vi "push.vi"() -> ()   [LabVIEW 2010]
panel:
  in  "stop":bool
  in  "OME string":string
  in  "notebook string":string
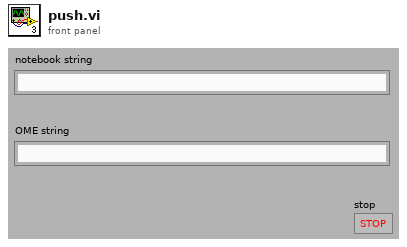
[diagram p1: front panel]
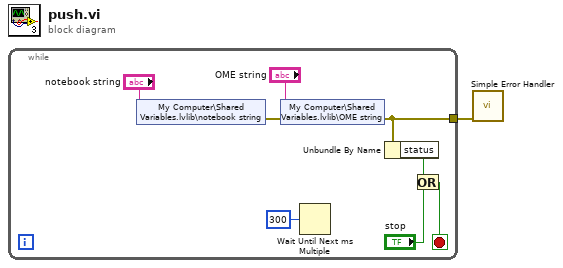
[diagram p0: block diagram]
diagram:
  n1 = while {
    tunnel: [w2] -> w1
    stop <- w3 stop-if-true
    n2 = shared-variable "My Computer\\Shared Variables.lvlib\\notebook string"("notebook string") -> (error out=w6:errorcluster)  [unwired: 1 in]
    n3 = shared-variable "My Computer\\Shared Variables.lvlib\\OME string"("OME string", error in=w6) -> (error out=w2:errorcluster)
    n4 = Wait Until Next ms Multiple(millisecond multiple=u32 300) -> ()  [unwired: 1 out]
    n5 = Unbundle By Name(w2) -> ("status"=w5:bool)
    n6 = Or(x=w5, y="stop") -> (x .or. y?=w3:bool)
  }
  n7 = call <vilib>:"Simple Error Handler.vi"("error in (no error)"=w1) -> ()  [unwired: 4 in, 5 out]
